vi "Normalized L-STF Cross Correlation.vi"(9 "input valid":bool, 10 "sample":T2) -> (1 "output valid":bool, 2 "normalized cross correlation":T1)   [LabVIEW 2020]
uses:
  <vilib>/rvi/IPIntegrationNode/IPINode_Typedef/niFpgaIPINodeSupportedFamilies.ctl
  <vilib>/rvi/FXPMathLib/FxpDiv/subVIs/nifxpmath_Div_SimConfig.ctl
  <vilib>/rvi/FXPMathLib/FxpSqrt/subVIs/nifxpmath_Sqrt_SimConfig.ctl
  <vilib>/fxp/LVFixedPointOverflowPolicyTypeDef.ctl
  <vilib>/rvi/FXPMathLib/FxpDiv/simVIs/DllFxpDivTemp_sub.vi
  <vilib>/rvi/IPIntegrationNode/IPINode_Utilities/niFpgaIPINodeSimCore.vi
  <vilib>/rvi/Emulation/niFpgaEmulationIsFPGAContextNoSignature.vi
  <vilib>/rvi/Emulation/niFpgaSctlEmulationGetInTimedLoop.vi
  <vilib>/rvi/errors/niFpgaSetErrorForExecOnDevCompSimple.vi
  <vilib>/rvi/eio/common/nirviEmuReportErrorAndStop.vi
  <vilib>/rvi/DataTransferAndStorage/Container/Common/niFpgaContainerGetUniqueNameForEmu.vi
  <vilib>/rvi/FIFO/Fifo_Resource/nirvififoEmulationSetSize.vi
  <vilib>/rvi/FIFO/Fifo_Resource/nirviFifoEmulationQueueMgr.vi
  <instcachedir>/0/nirviFifoEmulationQueueMgr_E5CAEC123FF24DC58D834DCA3CDAA9B5.lvgen/nirviFifoEmulationQueueMgr_E5CAEC123FF24DC58D834DCA3CDAA9B5_009.vi
  <vilib>/Utility/error.llb/Clear Errors.vi
  <vilib>/rvi/FIFO/Fifo_Resource/nirvififoEmulationCreateLock.vi
  <vilib>/rvi/Emulation/niFpgaProcessEmulError.vi
  <vilib>/rvi/FIFO/Fifo_Resource/nirvififoEmulationObtainLock.vi
  <vilib>/rvi/FIFO/Fifo_Resource/nirvififoEmulationReleaseLock.vi
  <vilib>/rvi/occurrence/nirviWaitOnOccurrenceBase.vi
  <vilib>/rvi/errors/nirviReportUnexpectedCaseInternalError.vi
  <vilib>/rvi/errors/nirviReportUnexpectedCaseInternalError (U32).vi
  <vilib>/rvi/FXPMathLib/FxpSqrt/simVIs/DllSqrtTemp_sub.vi
  <vilib>/rvi/FIFO/Fifo_Resource/nirvififoEmulationDetermineInputValidOut.vi
  <vilib>/rvi/FXPMathLib/FxpDiv/XNode/nifxpmath_Div.xnode
  <vilib>/rvi/XilinxIP/XIPIN_XNode/niFpgaXIPIN.xnode
  Normalized L-STF Cross Correlation/FIR Compiler 1/xsim.dir/FIR_Compiler_1_5AF33709C4C34337BEC33909FB17B7AF/xsimk_5AF33709C4C34337BEC33909FB17B7AF.dll
  <vilib>/rvi/IPIntegrationNode/IPINode_Xnode/niFpgaIPINode.xnode
  <vilib>/rvi/DataTransferAndStorage/Container/XNode/niFpgaContainer.xnode
  <vilib>/rvi/FIFO/Fifo_Resource/nirvififoEmulationRead.vi
  Normalized L-STF Cross Correlation/FIR Compiler/xsim.dir/FIR_Compiler_F9A70D62BDE24CE3A3A310E100390859/xsimk_F9A70D62BDE24CE3A3A310E100390859.dll
  <vilib>/rvi/FXPMathLib/FxpSqrt/XNode/nifxpmath_Sqrt.xnode
  <vilib>/rvi/FIFO/Fifo_Resource/nirvififoEmulationWrite.vi
types:
  T1 = cluster{"Real":fxp<+/-,18,1>, "Imag":fxp<+/-,18,1>}
  T2 = cluster{"Real":fxp<+/-,16,3>, "Imag":fxp<+/-,16,3>}
  T3 = cluster{"Real":fxp<+/-,37,10>, "Imag":fxp<+/-,37,10>}
  T4 = cluster{"Real":fxp<+/-,33,7>, "Imag":fxp<+/-,33,7>}
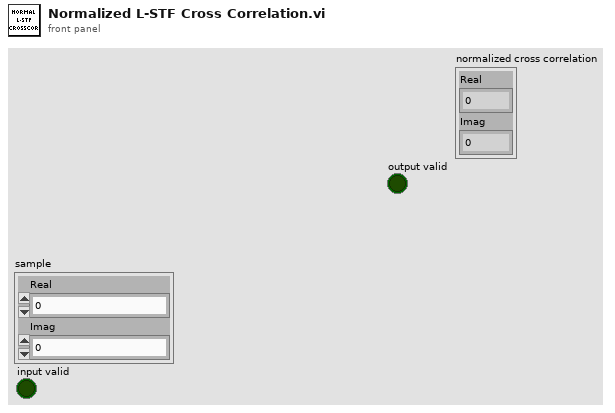
[diagram p1: front panel]
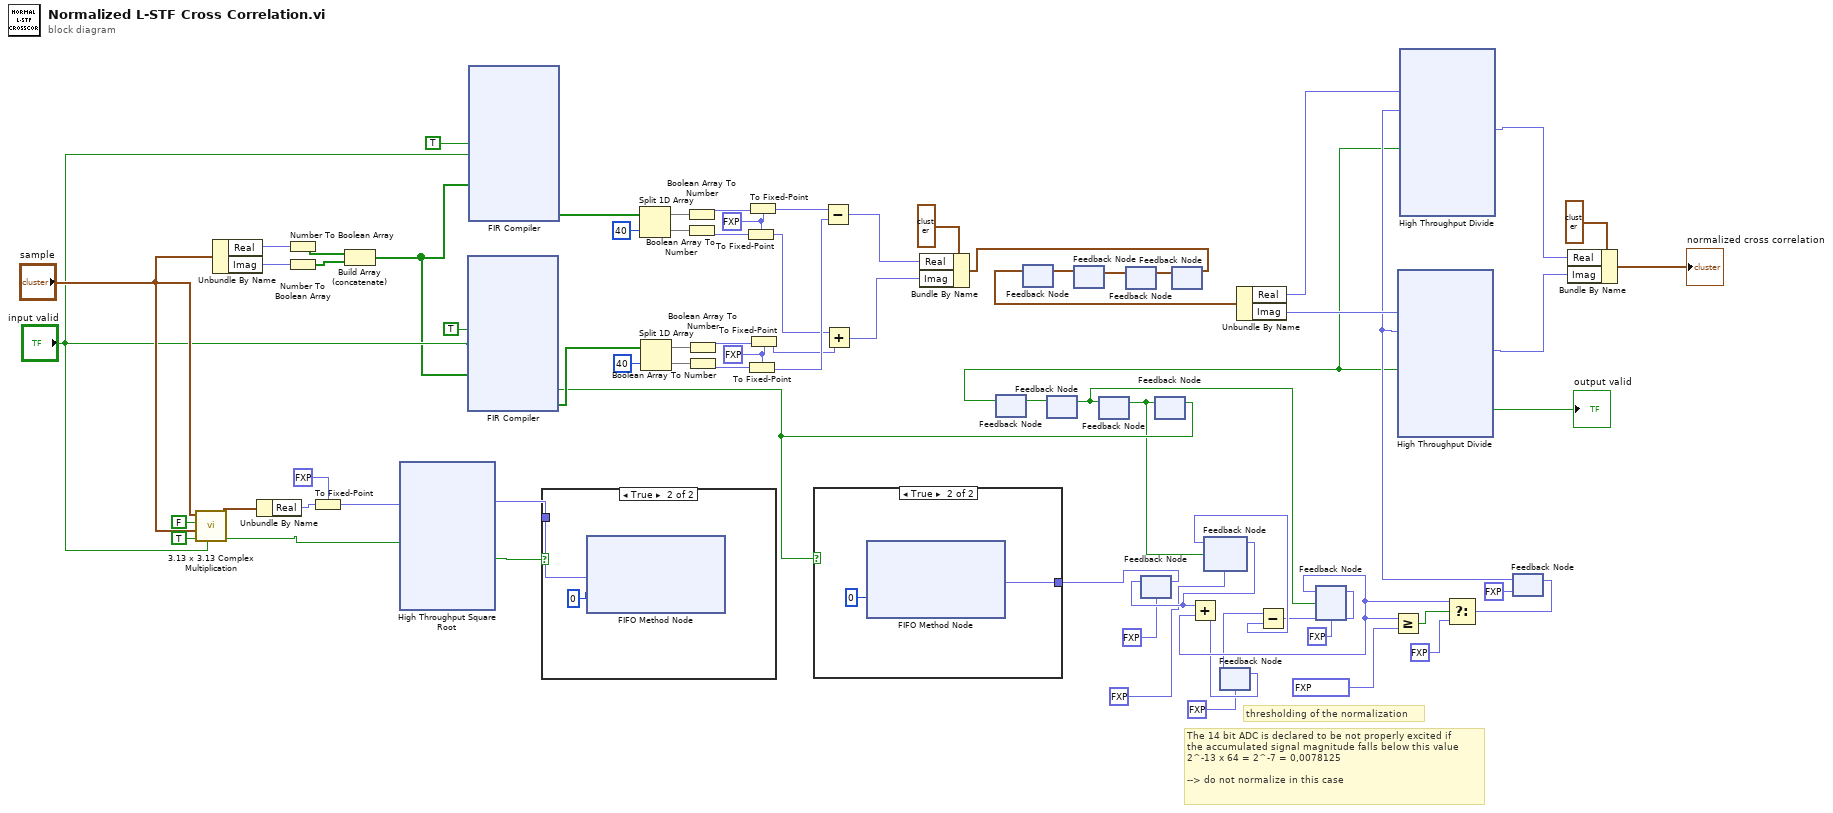
[diagram p0: block diagram]
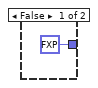
[diagram p2: hidden frame]
diagram:
  w44 = fxp<+/-,36,9> 0.0 ("fixed-point type")
  w51 = fxp<+/-,36,9> 0.0 ("fixed-point type")
  # "The 14 bit ADC is declared to be not properly excited if \nthe accumulated signal magnitude falls below this value\n2^-13 x 64 = 2^-7 = 0,0078125\n\n--> do not normalize in this case"
  # "thresholding of the normalization"
  n1 = call "3.13 x 3.13 Complex Multiplication.vi"("input valid"="input valid", "conjugate B"=TRUE, "B"="sample", "conjugate A"=FALSE, "A"="sample") -> ("output valid"=w67:bool, "product"=w71:T4)  [unwired: 5 in]
  n2 = Unbundle By Name("sample") -> ("Real"=w63:fxp<+/-,16,3>, "Imag"=w62:fxp<+/-,16,3>)
  n3 = Unbundle By Name(w71) -> ("Real"=w69:fxp<+/-,33,7>)
  n4 = Number To Boolean Array(number=w63) -> (Boolean array=w61:bool[])
  n5 = Number To Boolean Array(number=w62) -> (Boolean array=w60:bool[])
  n6 = To Fixed-Point(fixed-point type=fxp<+,32,6> 0.0, number=w69) -> (fixed-point=w68:fxp<+,32,6>)
  n7 = Build Array (concatenate)(w61, w60) -> (w56:bool[])
  n8 = xnode "High Throughput Square Root"("x"=w68, "input valid"=w67) -> ("sqrt(x)"=w65:fxp<+,16,3>, "output valid"=w66:bool)  [unwired: 1 in, 1 out]
  n9 = xnode ("FIR Compiler")("aclken"=TRUE, "s_axis_data_tvalid"="input valid", "s_axis_data_tdata"=w56) -> ("m_axis_data_tvalid"=w30:bool, "m_axis_data_tdata"=w42:bool[])  [unwired: 1 out]
  n10 = xnode ("FIR Compiler")("aclken"=TRUE, "s_axis_data_tvalid"="input valid", "s_axis_data_tdata"=w56) -> ("m_axis_data_tdata"=w50:bool[])  [unwired: 2 out]
  n11 = case shown="True" w66 {
    tunnel: w65 -> [_ w75]
    frame False {
    }
    frame True {
      n12 = xnode ("FIFO Method Node")("Element"=w75, "Timeout"=0) -> ()  [unwired: 1 in, 2 out]
    }
  }
  n13 = Split 1D Array(array=w50, index=40) -> (first subarray=w54:bool[], second subarray=w53:bool[])
  n14 = Split 1D Array(array=w42, index=40) -> (first subarray=w47:bool[], second subarray=w46:bool[])
  n15 = Boolean Array To Number(Boolean array=w54) -> (number=w49:fxp<+/-,40,13>)
  n16 = Boolean Array To Number(Boolean array=w53) -> (number=w52:fxp<+/-,40,13>)
  n17 = Boolean Array To Number(Boolean array=w47) -> (number=w43:fxp<+/-,40,13>)
  n18 = Boolean Array To Number(Boolean array=w46) -> (number=w45:fxp<+/-,40,13>)
  n19 = To Fixed-Point(fixed-point type=w51, number=w52) -> (fixed-point=w38:fxp<+/-,36,9>)
  n20 = To Fixed-Point(fixed-point type=w44, number=w45) -> (fixed-point=w40:fxp<+/-,36,9>)
  n21 = To Fixed-Point(fixed-point type=w51, number=w49) -> (fixed-point=w41:fxp<+/-,36,9>)
  n22 = To Fixed-Point(fixed-point type=w44, number=w43) -> (fixed-point=w39:fxp<+/-,36,9>)
  n23 = case shown="True" w30 {
    tunnel: [fxp<+,16,3> 0.0 ("Element") w77] -> w25
    frame False {
    }
    frame True {
      n24 = xnode ("FIFO Method Node")("Timeout"=0) -> ("Element"=w77:fxp<+,16,3>)  [unwired: 1 in, 2 out]
    }
  }
  n25 = Subtract(x=w41, y=w40) -> (x-y=w36:fxp<+/-,37,10>)
  n26 = Add(x=w38, y=w39) -> (x+y=w35:fxp<+/-,37,10>)
  n27 = Bundle By Name(cluster=T3 {"Real"=0.0, "Imag"=0.0} ("Complex"), "Real"=w36, "Imag"=w35) -> (w29:T3)
  n28 = feedback #1() -> (w10:bool)  [unwired: 1 in]
  n29 = feedback #2() -> (w28:T3)  [unwired: 1 in]
  n30 = feedback #3() -> (w31:bool)  [unwired: 1 in]
  n31 = feedback-in #1(w31) -> ()
  n32 = feedback #4() -> (w34:T3)  [unwired: 1 in]
  n33 = feedback-in #2(w34) -> ()
  n34 = feedback #5() -> (w6:bool)  [unwired: 1 in]
  n35 = feedback-in #3(w6) -> ()
  n36 = feedback #6() -> (w33:T3)  [unwired: 1 in]
  n37 = feedback-in #4(w33) -> ()
  n38 = feedback #7(fxp<+,22,9> 0.0) -> (w23:fxp<+,22,9>)
  n39 = feedback-in #7(w25) -> ()
  n40 = feedback #8() -> (w24:bool)  [unwired: 1 in]
  n41 = feedback-in #5(w24) -> ()
  n42 = feedback-in #8(w30) -> ()
  n43 = feedback #9() -> (w32:T3)  [unwired: 1 in]
  n44 = feedback-in #6(w32) -> ()
  n45 = feedback-in #9(w29) -> ()
  n46 = feedback #10(fxp<+,22,9> 0.0) -> (w22:fxp<+,22,9>)
  n47 = feedback-in #10(w23, w24) -> ()
  n48 = feedback #11(fxp<+,22,9> 0.0 ("x+y")) -> (w8:fxp<+,22,9>)
  n49 = Unbundle By Name(w28) -> ("Real"=w27:fxp<+/-,37,10>, "Imag"=w26:fxp<+/-,37,10>)
  n50 = Subtract(x=w8, y=w22) -> (x-y=w21:fxp<+,22,9>)
  n51 = feedback #12(fxp<+,22,9> 0.0) -> (w19:fxp<+,22,9>)
  n52 = Add(x=w23, y=w19) -> (x+y=w7:fxp<+,22,9>)
  n53 = feedback-in #11(w7) -> ()
  n54 = feedback-in #12(w21, w6) -> ()
  n55 = Greater Or Equal?(x=w19, y=fxp<+/-,22,9> 0.0078125) -> (x >= y?=w20:bool)
  n56 = Select(t=w19, s=w20, f=fxp<+,22,9> 1.0) -> (s? t:f=w16:fxp<+,22,9>)
  n57 = feedback #13(fxp<+,22,9> 0.0 ("f")) -> (w15:fxp<+,22,9>)
  n58 = xnode "High Throughput Divide"("x"=w26, "y"=w15, "input valid"=w10) -> ("x/y"=w12:fxp<+/-,18,1>, "output valid"=→"output valid":bool)  [unwired: 1 in, 1 out]
  n59 = xnode "High Throughput Divide"("x"=w27, "y"=w15, "input valid"=w10) -> ("x/y"=w13:fxp<+/-,18,1>)  [unwired: 1 in, 2 out]
  n60 = feedback-in #13(w16) -> ()
  n61 = Bundle By Name(cluster=T1 {"Real"=0.0, "Imag"=0.0} ("Complex"), "Real"=w13, "Imag"=w12) -> (→"normalized cross correlation":T1)
